vi "Digital In Test_TS.vi"(8 "error in (no error)":errorcluster, 10 "Message IN":string) -> (0 "error out":errorcluster, 1 "Result (bool)":bool, 2 "Message OUT":string, 3 "VISA OUT":refnum<visa-resource-name>)   [LabVIEW 2022 SP3]
uses:
  <vilib>/DAQmx/write.llb/DAQmx Write (Digital 1D Bool NChan 1Samp 1Line).vi
  <vilib>/DAQmx/miscellaneous.llb/DAQmx Fill In Error Info.vi
panel:
  out "cDAQ DO Cmd":bool[](array[boolean])
  out "DI Reading":bool[](array[boolean])
  out "Result (color)":u32(colorbox)
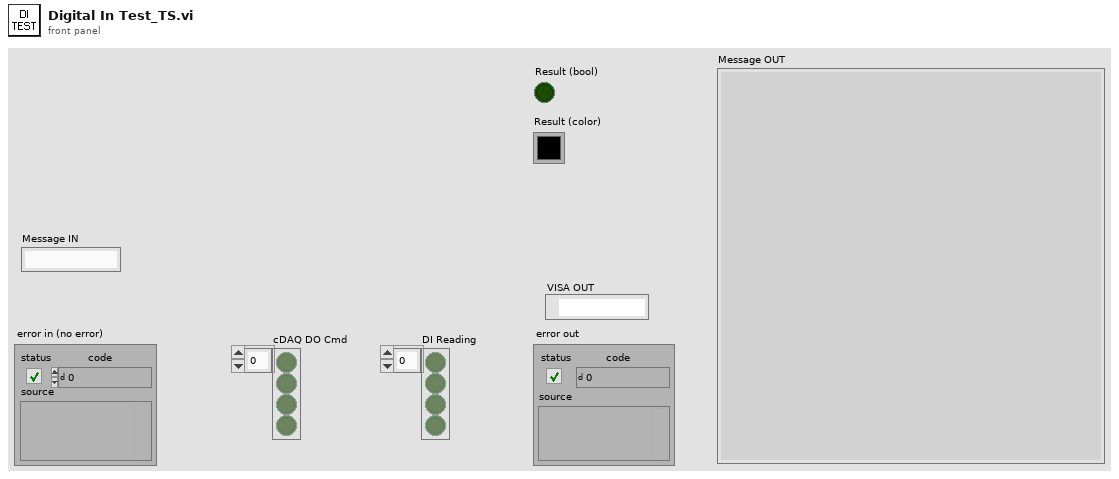
[diagram p1: front panel]
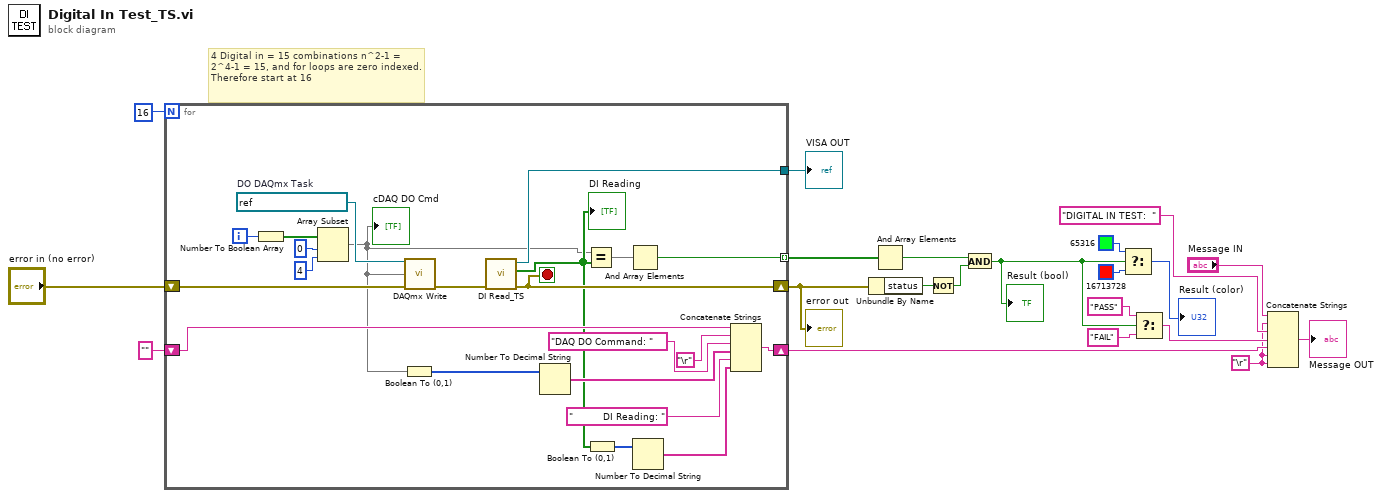
[diagram p0: block diagram]
diagram:
  w5 = "\r"
  # "4 Digital in = 15 combinations n^2-1 = 2^4-1 = 15, and for loops are zero indexed.  Therefore start at 16"
  n1 = for {
    N: 16 -> [_]
    shift-right: [w37] -> w2
    shift-left: "error in (no error)" -> [w43]
    tunnel: [w42] -> w3
    tunnel: [w41] -> w15 mode=indexing
    shift-right: [w29] -> w10
    shift-left: "" -> [w28]
    i -> [w38]
    stop <- w37 stop-if-true
    w39 = refnum<k21> "FTS2_DigitalOut"  # DO DAQmx Task
    n2 = Number To Boolean Array(number=w38) -> (Boolean array=w23:bool[])
    n3 = Array Subset(array=w23, index=0, length=4) -> (w24:bool[])
    "cDAQ DO Cmd" <- w24
    n4 = Boolean To (0,1)(Boolean=w24) -> (0, 1=w31:i16[])
    n5 = call-poly <vilib>:"DAQmx Write.vi"("task/channels in"=w39, "data"=w24, "error in"=w43) -> ("error out"=w22:errorcluster)  [unwired: 10 in, 2 out]
    n6 = call "DI Read_TS.vi"("error in (no error)"=w22) -> ("error out"=w37:errorcluster, "DI Reading"=w27:bool[], "VISA Refnum out"=w42:refnum<visa-resource-name>)  [unwired: 7 in, 1 out]
    "DI Reading" <- w27
    n7 = Number To Decimal String(number=w31) -> (decimal integer string=w34:string[])  [unwired: 1 in]
    n8 = Equal?(x=w24, y=w27) -> (x = y?=w40:bool[])
    n9 = Boolean To (0,1)(Boolean=w27) -> (0, 1=w30:i16[])
    n10 = And Array Elements(Boolean array=w40) -> (logical AND=w41:bool)
    n11 = Number To Decimal String(number=w30) -> (decimal integer string=w36:string[])  [unwired: 1 in]
    n12 = Concatenate Strings(w28, "\r", "DAQ DO Command: ", w34, "          DI Reading: ", w36) -> (w29:string)
  }
  "error out" <- w2
  "VISA OUT" <- w3
  n13 = Unbundle By Name(w2) -> ("status"=w14:bool)
  n14 = And Array Elements(Boolean array=w15) -> (logical AND=w12:bool)
  n15 = Not(x=w14) -> (.not. x?=w11:bool)
  n16 = And(x=w12, y=w11) -> (x .and. y?=w13:bool)
  "Result (bool)" <- w13
  n17 = Select(t=u32 65316 ("Result (color)"), s=w13, f=u32 16713728 ("Result (color)")) -> (s? t:f=→"Result (color)":u32)
  n18 = Select(t="PASS", s=w13, f="FAIL") -> (s? t:f=w7:string)
  n19 = Concatenate Strings("Message IN", w5, "DIGITAL IN TEST:  ", w7, w10, w5, w5) -> (→"Message OUT":string)
